vi "Round.vi"(11 "Number":dbl) -> (3 "Rounded number":i32)   [LabVIEW 2010]
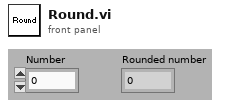
[diagram p1: front panel]
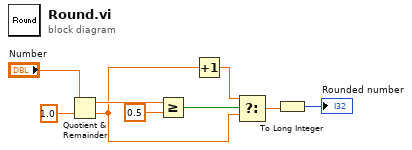
[diagram p0: block diagram]
diagram:
  n1 = Quotient & Remainder(x="Number", y=1.0) -> (x-y*floor(x/y)=w7:dbl, floor(x/y)=w3:dbl)
  n2 = Greater Or Equal?(x=w7, y=0.5) -> (x >= y?=w5:bool)
  n3 = Increment(x=w3) -> (x+1=w4:dbl)
  n4 = Select(t=w4, s=w5, f=w3) -> (s? t:f=w2:dbl)
  n5 = To Long Integer(number=w2) -> (32bit integer=→"Rounded number":i32)
